vi "Agilent 4194 Measure Impedance.vi"() -> ()   [LabVIEW 2010]
doc: "This function illustrates sample measurement of impedance and returns the average measured data of both measured parameters.\n\nNotes:\n\nThis example demonstrates the only way how to use this instrument driver."
uses:
  <instrlib>/Agilent 4194/Agilent 4194.lvlib
panel:
  in  "VISA resource name":refnum<visa-resource-name>
  in  "error in (no error)":errorcluster
  out "Average Line Cursor Value B":dbl format="%^.3e"
  out "Average Line Cursor Value A":dbl format="%^.3e"
  in  "Impedance (0:| Z | - theta)":u32(ring) items=["| Z | - theta ", "R - X", "Ls-Rs", "Ls-Q", "Cs-Rs", "Cs-Q", "Cs-D", "|Y|-theta", "G-B", "Lp-G", "Lp-Q", "Cp-G", "Cp-Q", "Cp-D", "|Z|-Ls", "|Z|-Cs", "|Z|-Lp", "|Z|-Cp", "Lp-Rp", "Cp-Rp"]
  # "© 2005 National Instruments.  ALL RIGHTS RESERVED."
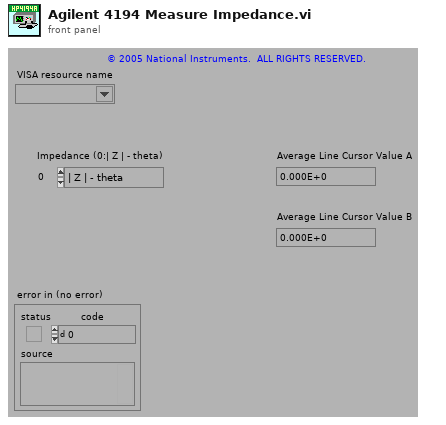
[diagram p1: front panel]
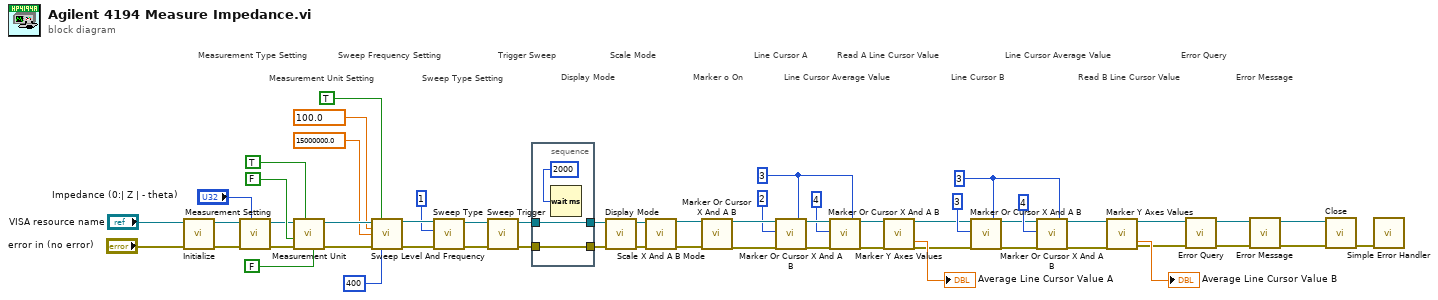
[diagram p0: block diagram]
diagram:
  w24 = u32 3 ("Marker/Line Cursor (1:o Marker On)")
  w31 = u32 3 ("Marker/Line Cursor (1:o Marker On)")
  # "Error Message"
  # "Error Query"
  # "Line Cursor B"
  # "Line Cursor Average Value"
  # "Read B Line Cursor Value"
  # "Read A Line Cursor Value"
  # "Line Cursor Average Value"
  # "Line Cursor A"
  # "Marker o On"
  # "Scale Mode"
  # "Display Mode"
  # "Trigger Sweep"
  # "Sweep Type Setting"
  # "Sweep Frequency Setting"
  # "Measurement Unit Setting"
  # "Measurement Type Setting"
  n1 = call <instrlib>:"Initialize.vi"("error in (no error)"="error in (no error)", "VISA resource name"="VISA resource name") -> ("error out"=w7:errorcluster, "VISA resource name out"=w6:refnum<visa-resource-name>)  [unwired: 8 in]
  n2 = call <instrlib>:"Measurement Setting.vi"("Measurement Type (0:Impedance)"="Impedance (0:| Z | - theta)", "error in (no error)"=w7, "VISA resource name"=w6) -> ("error out"=w52:errorcluster, "VISA resource name out"=w53:refnum<visa-resource-name>)  [unwired: 7 in]
  n3 = call <instrlib>:"Measurement Unit.vi"("Test Input Impedance(T:50 ohm)"=FALSE ("Ref Attenuation (F:0 dB)"), "Power Splitter (F:Dual)"=TRUE ("Ref Attenuation (F:0 dB)"), "error in (no error)"=w52, "Ref Input Impedance (T:50 ohm)"=FALSE ("Ref Attenuation (F:0 dB)"), "VISA resource name"=w53) -> ("error out"=w49:errorcluster, "VISA resource name out"=w50:refnum<visa-resource-name>)  [unwired: 5 in]
  n4 = call <instrlib>:"Sweep Level And Frequency.vi"("VISA resource name"=w50, "Step/Number Of Points (F:Points)"=TRUE ("Step/Number Of Points (F:Points))"), "Start/Center (10,00E-3)"=100.0 ("Stop/Span (10,00E-3)"), "Stop/Span (10,00E-3)"=15000000.0, "error in (no error)"=w49, "Number Of Points (100)"=400) -> ("VISA resource name out"=w44:refnum<visa-resource-name>, "error out"=w43:errorcluster)  [unwired: 8 in]
  n5 = call <instrlib>:"Sweep Type.vi"("error in (no error)"=w43, "Sweep Mode (0:Repeat)"=u32 1, "VISA resource name"=w44) -> ("error out"=w40:errorcluster, "VISA resource name out"=w41:refnum<visa-resource-name>)  [unwired: 7 in]
  n6 = call <instrlib>:"Sweep Trigger.vi"("error in (no error)"=w40, "VISA resource name"=w41) -> ("error out"=w15:errorcluster, "VISA resource name out"=w14:refnum<visa-resource-name>)  [unwired: 8 in]
  n7 = stacked-sequence {
    tunnel: w15 -> [w58]
    tunnel: [w59] -> w13
    tunnel: w14 -> [w59]
    tunnel: [w58] -> w12
    frame #0 {
      n8 = Wait (ms)(milliseconds to wait=u32 2000) -> ()  [unwired: 1 out]
    }
  }
  n9 = call <instrlib>:"Display Mode.vi"("error in (no error)"=w12, "VISA resource name"=w13) -> ("error out"=w38:errorcluster, "VISA resource name out"=w39:refnum<visa-resource-name>)  [unwired: 8 in]
  n10 = call <instrlib>:"Scale X And A B Mode.vi"("VISA resource name"=w39, "error in (no error)"=w38) -> ("VISA resource name out"=w37:refnum<visa-resource-name>, "error out"=w36:errorcluster)  [unwired: 12 in]
  n11 = call <instrlib>:"Marker Or Cursor X And A B.vi"("VISA resource name"=w37, "error in (no error)"=w36) -> ("VISA resource name out"=w34:refnum<visa-resource-name>, "error out"=w33:errorcluster)  [unwired: 16 in]
  n12 = call <instrlib>:"Marker Or Cursor X And A B.vi"("VISA resource name"=w34, "LMark/oMark/LCurs(0:Line Curs)"=u32 2 ("L Mark/o Mark and L Cursor (0:Line curs val)"), "error in (no error)"=w33, "Marker/LineCurs(1:oMarker On)"=w31) -> ("VISA resource name out"=w35:refnum<visa-resource-name>, "error out"=w28:errorcluster)  [unwired: 14 in]
  n13 = call <instrlib>:"Marker Or Cursor X And A B.vi"("VISA resource name"=w35, "LMark/oMark/LCurs(0:Line Curs)"=u32 4 ("L Mark/o Mark and L Cursor (0:Line curs val)"), "error in (no error)"=w28, "Marker/LineCurs(1:oMarker On)"=w31) -> ("VISA resource name out"=w29:refnum<visa-resource-name>, "error out"=w27:errorcluster)  [unwired: 14 in]
  n14 = call <instrlib>:"Marker Y Axes Values.vi"("VISA resource name"=w29, "error in (no error)"=w27) -> ("VISA resource name out"=w22:refnum<visa-resource-name>, "Line Curs Value"=→"Average Line Cursor Value A":dbl, "error out"=w19:errorcluster)  [unwired: 6 in, 9 out]
  n15 = call <instrlib>:"Marker Or Cursor X And A B.vi"("VISA resource name"=w22, "LMark/oMark/LCurs(0:Line Curs)"=u32 3 ("L Mark/o Mark and L Cursor (0:Line curs val)"), "error in (no error)"=w19, "Marker/LineCurs(1:oMarker On)"=w24) -> ("VISA resource name out"=w21:refnum<visa-resource-name>, "error out"=w18:errorcluster)  [unwired: 14 in]
  n16 = call <instrlib>:"Marker Or Cursor X And A B.vi"("VISA resource name"=w21, "LMark/oMark/LCurs(0:Line Curs)"=u32 4 ("L Mark/o Mark and L Cursor (0:Line curs val)"), "error in (no error)"=w18, "Marker/LineCurs(1:oMarker On)"=w24) -> ("VISA resource name out"=w20:refnum<visa-resource-name>, "error out"=w17:errorcluster)  [unwired: 14 in]
  n17 = call <instrlib>:"Marker Y Axes Values.vi"("VISA resource name"=w20, "error in (no error)"=w17) -> ("VISA resource name out"=w11:refnum<visa-resource-name>, "Line Curs Value"=→"Average Line Cursor Value B":dbl, "error out"=w9:errorcluster)  [unwired: 6 in, 9 out]
  n18 = call <instrlib>:"Error Query.vi"("error in (no error)"=w9, "VISA resource name"=w11) -> ("error out"=w8:errorcluster, "VISA resource name out"=w10:refnum<visa-resource-name>)  [unwired: 6 in, 2 out]
  n19 = call <instrlib>:"Error Message.vi"("error in (no error)"=w8, "VISA resource name"=w10) -> ("error out"=w2:errorcluster, "VISA resource name out"=w3:refnum<visa-resource-name>)  [unwired: 5 in, 3 out]
  n20 = call <instrlib>:"Close.vi"("error in (no error)"=w2, "VISA resource name"=w3) -> ("error out"=w1:errorcluster)  [unwired: 9 in]
  n21 = call <vilib>:"Simple Error Handler.vi"("error in (no error)"=w1) -> ()  [unwired: 4 in, 5 out]
